vi "Model_Info_and_Report_Write_Eval_Layer_Info.vi"(5 "Evaluation_Metrics":T3 {"Evaluation_Metrics(Image)"."Eval Stats"."Recall(F1_Max)" format="%#.5f"; "Evaluation_Metrics(Image)"."Eval Stats"."FPR(F1_Max)" format="%#.5f"; "Evaluation_Metrics(Image)"."Eval Stats"."FNR(F1_Max)" format="%#.5f"; "Evaluation_Metrics(Image)"."Eval Stats"."Prec.(F1_Max)" format="%#.5f"; "Evaluation_Metrics(Image)"."Eval Stats"."F1_Max" format="%#.5f"; "Evaluation_Metrics(Image)"."Eval Stats"."AUROC" format="%#.5f"; "Evaluation_Metrics(Image)"."Eval Stats"."Scores(Bad)"."Min" format="%#_5g"; "Evaluation_Metrics(Image)"."Eval Stats"."Scores(Good)"."Min" format="%#_5g"; "Evaluation_Metrics(Image)"."Eval Stats"."Thrshld(F1_Max)" format="%#_5f"; "Evaluation_Metrics(Pixel)"."Eval Stats"."Recall(F1_Max)" format="%#.5f"; "Evaluation_Metrics(Pixel)"."Eval Stats"."FPR(F1_Max)" format="%#.5f"; "Evaluation_Metrics(Pixel)"."Eval Stats"."FNR(F1_Max)" format="%#.5f"; "Evaluation_Metrics(Pixel)"."Eval Stats"."Prec.(F1_Max)" format="%#.5f"; "Evaluation_Metrics(Pixel)"."Eval Stats"."F1_Max" format="%#.5f"; "Evaluation_Metrics(Pixel)"."Eval Stats"."AUROC" format="%#.5f"; "Evaluation_Metrics(Pixel)"."Eval Stats"."Scores(Bad)"."Min" format="%#_5g"; "Evaluation_Metrics(Pixel)"."Eval Stats"."Scores(Good)"."Min" format="%#_5g"; "Evaluation_Metrics(Pixel)"."Eval Stats"."Thrshld(F1_Max)" format="%#_5f"}, 7 "[LayerID, PatchSize]":T1=[{"Layer_ID"=8, "Patch_Size"=3}, {"Layer_ID"=16, "Patch_Size"=3}], 11 "Model_Info_and_Report in":T2={"Idx"=0, "Name"="", "Feature Extractor"="wrn_50_2_2_bnmerge", "Layers"="", "DS_Size"=0, "H"=0, "W"=-1, "Coreset Size"=0, "Proj_Dim"=0, "Good_Max(Img)"=0.0, "Bad_Min(Img)"=0.0, "Rel_Margin"=0.0, "Image_AUC"=0.0, "Pixel_AUC"=0.0, "Image_F1_Max"=0.0, "Pixel_F1_Max"=0.0, "Train_Time"=0.0, "Inf_Time"=0.0} {"Rel_Margin" format="%#.5f"; "Bad_Min(Img)" format="%#.5f"; "Good_Max(Img)" format="%#.5f"; "Pixel_F1_Max" format="%#.5f"; "Pixel_AUC" format="%#.5f"; "Image_F1_Max" format="%#.5f"; "Image_AUC" format="%#.5f"}) -> (3 "Model_Info_and_Report out":T2={"Idx"=0, "Name"="", "Feature Extractor"="wrn_50_2_2_bnmerge", "Layers"="", "DS_Size"=0, "H"=-1, "W"=-1, "Coreset Size"=0, "Proj_Dim"=0, "Good_Max(Img)"=0.9999726, "Bad_Min(Img)"=0.9949659, "Rel_Margin"=0.9949659, "Image_AUC"=0.9999726, "Pixel_AUC"=0.9999726, "Image_F1_Max"=0.9949659, "Pixel_F1_Max"=0.9949659, "Train_Time"=0.0, "Inf_Time"=0.0} {"Rel_Margin" format="%#.5f"; "Bad_Min(Img)" format="%#.5f"; "Good_Max(Img)" format="%#.5f"; "Pixel_F1_Max" format="%#.5f"; "Pixel_AUC" format="%#.5f"; "Image_F1_Max" format="%#.5f"; "Image_AUC" format="%#.5f"})   [LabVIEW 2020]
uses:
  Controls/Model_Info_and_Report.ctl
  <vilib>/Ngene/DeepLTK Anomaly Detection Addon/Toolkit/API/Controls/Evaluation_Metrics(Pixel_Image).ctl
  <vilib>/Ngene/DeepLTK Anomaly Detection Addon/Toolkit/API/Controls/Evaluation_Metrics.ctl
  <vilib>/Ngene/DeepLTK Anomaly Detection Addon/Toolkit/API/Controls/Eval_Results.ctl
  <vilib>/Ngene/DeepLTK Anomaly Detection Addon/Toolkit/API/Controls/MinMax.ctl
  Controls/Feature_Layers_CFG.ctl
  <vilib>/Ngene/DeepLTK Anomaly Detection Addon/Toolkit/DeepLTK_Anomaly_Detection_Addon.lvlib
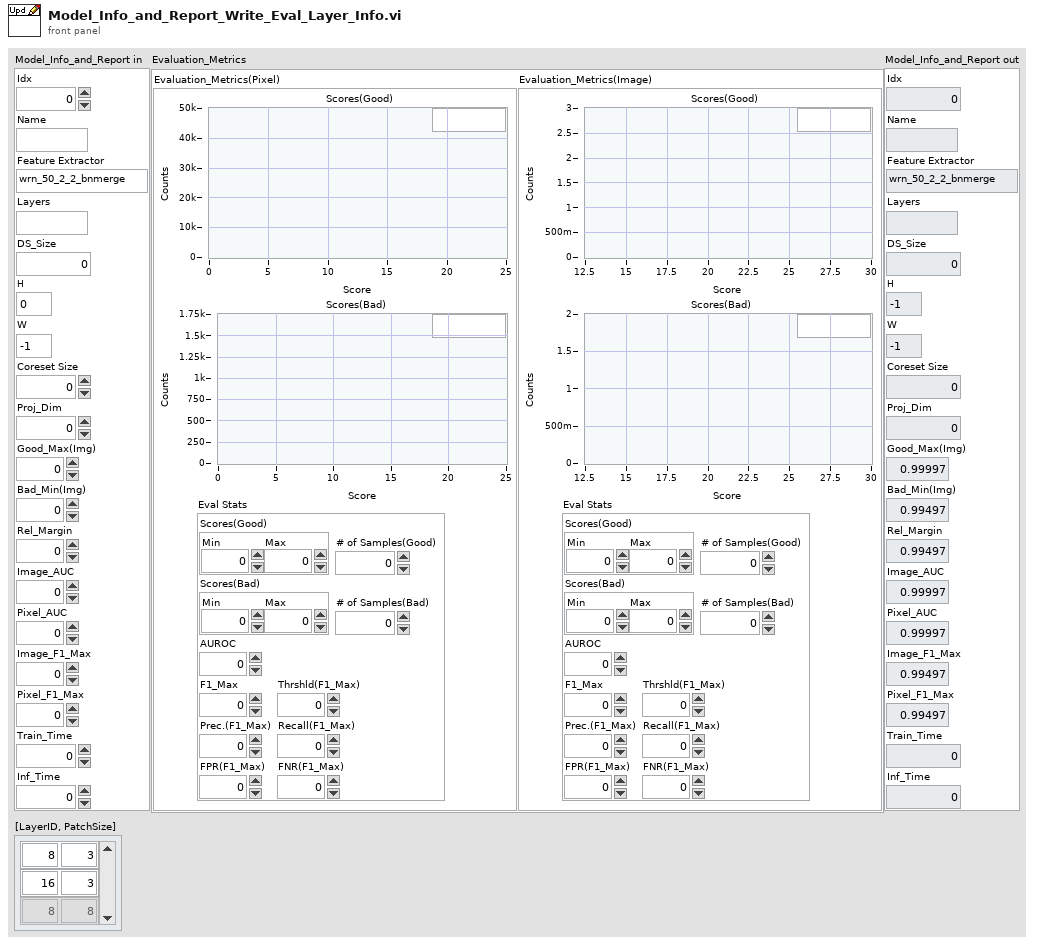
[diagram p1: front panel]
types:
  T1 = typedef "Feature_Layers_CFG.ctl" = cluster{"Layer_ID":i32, "Patch_Size":i32}[]
  T2 = typedef "Model_Info_and_Report.ctl" = cluster{"Idx":i32, "Name":string, "Feature Extractor":string, "Layers":string, "DS_Size":i32, "H":i32, "W":i32, "Coreset Size":i32, "Proj_Dim":i32, "Good_Max(Img)":sgl, "Bad_Min(Img)":sgl, "Rel_Margin":sgl, "Image_AUC":sgl, "Pixel_AUC":sgl, "Image_F1_Max":sgl, "Pixel_F1_Max":sgl, "Train_Time":dbl, "Inf_Time":dbl}
  T3 = typedef "DeepLTK_Anomaly_Detection_Addon.lvlib/Evaluation_Metrics(Pixel_Image).ctl" = cluster{"Evaluation_Metrics(Pixel)":T4, "Evaluation_Metrics(Image)":T4}
  T4 = typedef "DeepLTK_Anomaly_Detection_Addon.lvlib/Evaluation_Metrics.ctl" = cluster{"Scores(Good)":cluster{"X Values":dbl[], "Histogram: h(x)":i32[]}, "Scores(Bad)":cluster{"X Values":dbl[], "Histogram: h(x)":i32[]}, "Eval Stats":T5}
  T5 = typedef "DeepLTK_Anomaly_Detection_Addon.lvlib/Eval_Results.ctl" = cluster{"Scores(Good)":T6, "Scores(Bad)":T6, "# of Samples(Good)":i32, "# of Samples(Bad)":i32, "AUROC":sgl, "F1_Max":sgl, "Thrshld(F1_Max)":sgl, "Prec.(F1_Max)":sgl, "Recall(F1_Max)":sgl, "FPR(F1_Max)":sgl, "FNR(F1_Max)":sgl}
  T6 = typedef "DeepLTK_Anomaly_Detection_Addon.lvlib/MinMax.ctl" = cluster{"Min":sgl, "Max":sgl}
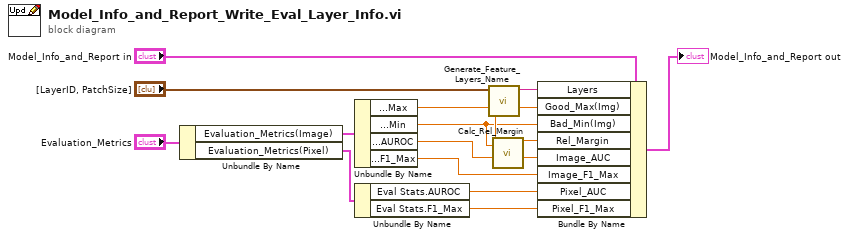
[diagram p0: block diagram]
diagram:
  n1 = Unbundle By Name("Evaluation_Metrics") -> ("Evaluation_Metrics(Image)"=w11:T4, "Evaluation_Metrics(Pixel)"=w3:T4)
  n2 = Unbundle By Name(w11) -> ("Eval Stats.Scores(Good).Max"=w14:sgl, "Eval Stats.Scores(Bad).Min"=w13:sgl, "Eval Stats.AUROC"=w10:sgl, "Eval Stats.F1_Max"=w9:sgl)
  n3 = Unbundle By Name(w3) -> ("Eval Stats.AUROC"=w8:sgl, "Eval Stats.F1_Max"=w7:sgl)
  n4 = call "Generate_Feature_Layers_Name.vi"("[LayerID, PatchSize]"="[LayerID, PatchSize]") -> ("Layers"=w6:string)  [unwired: 10 in]
  n5 = call "Calc_Rel_Margin.vi"("Max"=w14, "Min"=w13) -> ("Rel_Margin"=w12:sgl)  [unwired: 17 in]
  n6 = Bundle By Name(cluster="Model_Info_and_Report in", "Layers"=w6, "Good_Max(Img)"=w14, "Bad_Min(Img)"=w13, "Rel_Margin"=w12, "Image_AUC"=w10, "Image_F1_Max"=w9, "Pixel_AUC"=w8, "Pixel_F1_Max"=w7) -> (→"Model_Info_and_Report out":T2)
